vi "DB Tools Open Connection.vi"   [LabVIEW 2013, in "NI_Database_API_64.lvlib"]
doc: "Opens a database connection using the connection information path and returns a connection reference. If <B>prompt?</B> is set to TRUE, LabVIEW displays a dialog box to set up the connection. Wire data to the <B>connection information</B> input to determine the polymorphic instance to use or manually select the instance."
uses:
  NI_Database_API_64.lvlib
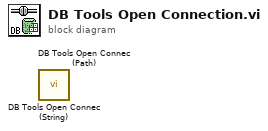
[diagram p0: block diagram]
diagram:
  n1 = call "DB Tools Open Connec (String).vi"() -> ()  [unwired: 8 in, 2 out]
  n2 = call "DB Tools Open Connec (Path).vi"() -> ()  [unwired: 8 in, 2 out]
